vi "Find Specify Color Index.vi"(6 "Color Box":u32(colorbox)=16776960, 7 "Num of Row":i32, 8 "error in (no error)":errorcluster, 10 "Column":i32, 11 "MultiList Ref In":refnum<vi>) -> (0 "error out":errorcluster, 1 "Index":i32, 3 "MultiList Ref Out":refnum<vi>, 4 "Exist?":bool, 5 "Active Cell":T1)   [LabVIEW 2019]
uses:
  <vilib>/Utility/miscctls.llb/LVRowAndColumnTypeDef.ctl
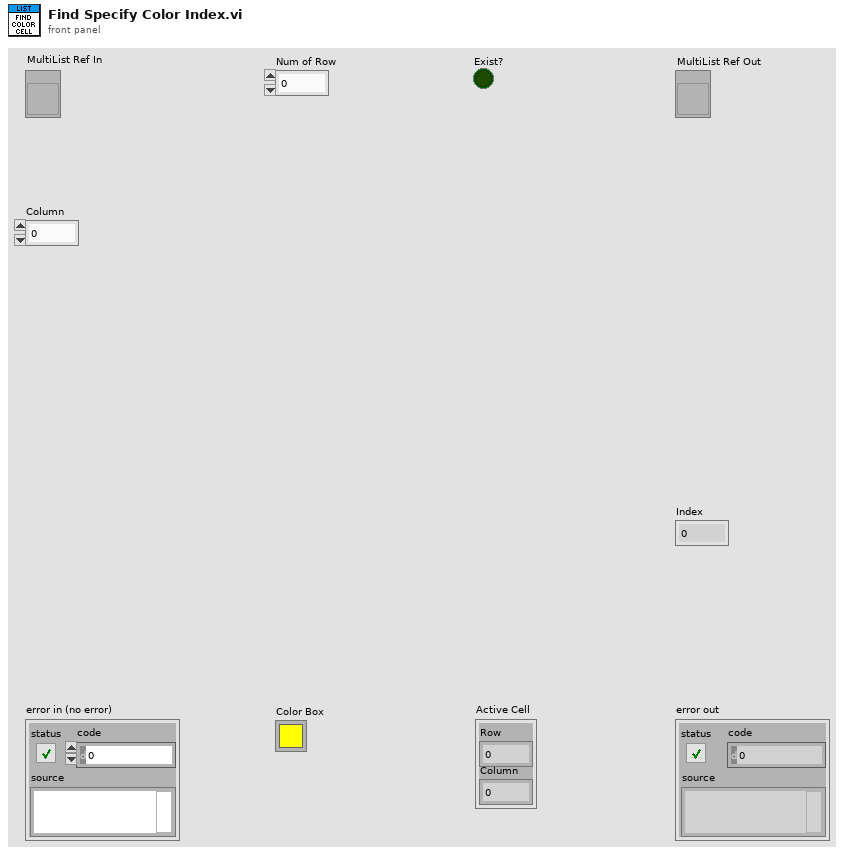
[diagram p1: front panel]
types:
  T1 = typedef "LVRowAndColumnTypeDef.ctl" = cluster{"Row":i32, "Column":i32}
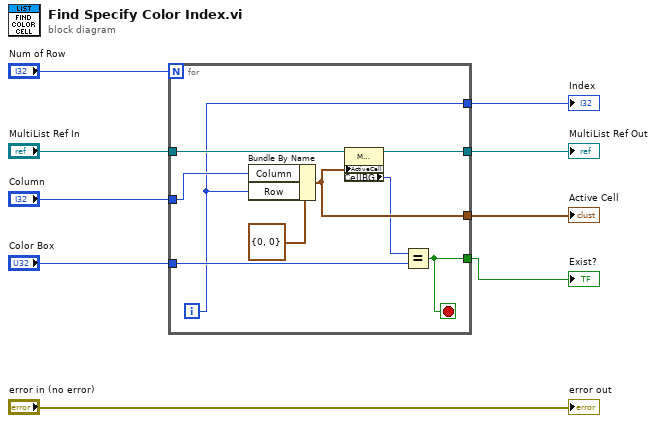
[diagram p0: block diagram]
diagram:
  n1 = for {
    N: "Num of Row" -> [_]
    tunnel: "MultiList Ref In" -> [w17]
    tunnel: "Column" -> [w16]
    tunnel: [w15] -> w7
    tunnel: "Color Box" -> [w14]
    tunnel: [w13] -> w6
    tunnel: [w12] -> w3
    tunnel: [w10] -> w2
    i -> [w10]
    stop <- w13 stop-if-true
    n2 = Bundle By Name(cluster=T1 {"Row"=0, "Column"=0} ("Active Cell:Active Cell"), "Column"=w16, "Row"=w10) -> (w15:T1)
    n3 = property class="MCListbox (strict)"(reference=w17, "ActiveCell"=w15) -> (reference out=w12:refnum<vi>, "CellBG"=w11:u32)  [unwired: 1 in, 1 out]
    n4 = Equal?(x=w11, y=w14) -> (x = y?=w13:bool)
  }
  "Active Cell" <- w7
  "Exist?" <- w6
  "MultiList Ref Out" <- w3
  "Index" <- w2
  "error out" <- "error in (no error)"
